vi "updateGoalAmount.vi"(8 "error in (no error)":errorcluster, 10 "Goal.lvclass":refnum<class "Goal.lvclass">, 11 "Database in":refnum<class "Account History.lvclass">) -> (0 "error out":errorcluster, 3 "Database out":refnum<class "Account History.lvclass">)   [LabVIEW 2018, in "Account History.lvclass"]
uses:
  Account History.lvclass
  Goal/Goal.lvclass
  C:/GitRepos/Filthy-Lucre-Budgetizer/source/support/classes/UserEditableAmount/UserEditableAmount.lvclass
  UserEditableAmount/UserEditableAmount.lvclass
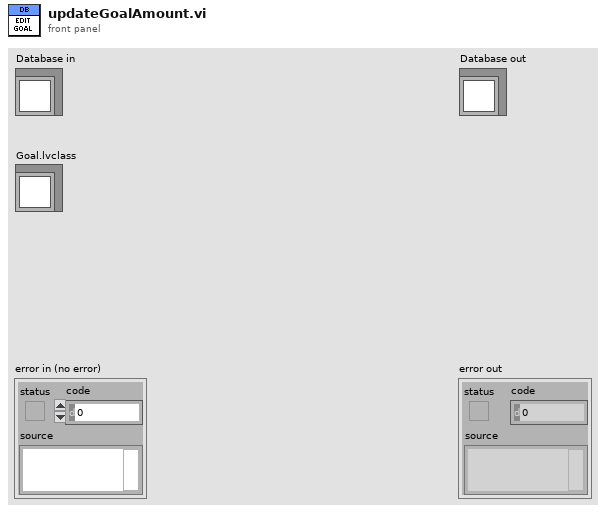
[diagram p1: front panel]
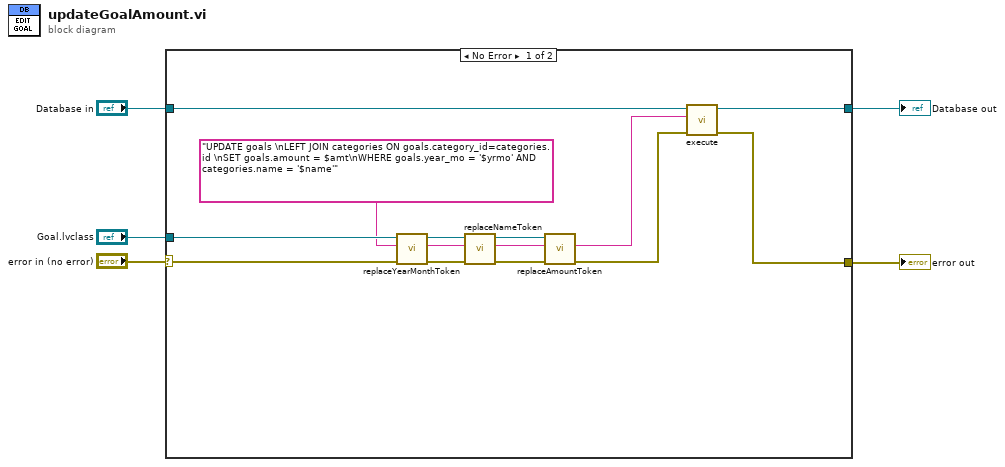
[diagram p0: block diagram]
diagram:
  n1 = case shown="No Error" "error in (no error)" {
    selector: "error in (no error)" -> [w14 w21]
    tunnel: [w17 w21] -> w4
    tunnel: [w18 w20] -> w2
    tunnel: "Database in" -> [w19 w20]
    tunnel: "Goal.lvclass" -> [w16 _]
    frame No Error {
      n2 = call "replaceYearMonthToken.vi"("error in (no error)"=w14, "Querry In"="UPDATE goals \nLEFT JOIN categories ON goals.category_id=categories.id \nSET goals.amount = $amt\nWHERE goals.year_mo = '$yrmo' AND categories.name = '$name'", "Goal in"=w16) -> ("error out"=w13:errorcluster, "Query Out"=w12:string, "Goal out"=w15:refnum<class "Goal.lvclass">)  [unwired: 6 in]
      n3 = call "replaceNameToken.vi"("error in (no error)"=w13, "Query In"=w12, "Goal in"=w15) -> ("error out"=w8:errorcluster, "Query Out"=w9:string, "Goal out"=w10:refnum<class "Goal.lvclass">)  [unwired: 6 in]
      n4 = call "replaceAmountToken.vi"("error in (no error)"=w8, "Query In"=w9, "UserEditableAmount in"=w10) -> ("error out"=w7:errorcluster, "Query Out"=w6:string)  [unwired: 6 in, 1 out]
      n5 = call "execute.vi"("error in (no error)"=w7, "SQL query"=w6, "Database in"=w19) -> ("error out"=w17:errorcluster, "Database out"=w18:refnum<class "Account History.lvclass">)  [unwired: 7 in]
    }
    frame Error {
    }
  }
  "error out" <- w4
  "Database out" <- w2
